vi "JKI_Python_Server - VI Tree.vi"   [LabVIEW 2013]
uses:
  Server/Server.lvclass
  Call/Call.lvclass
types:
  T1 = typedef "JKI_Python_Bridge_for_LV.lvlib/Server.lvclass/Python Method Call - Event Registration.ctl" = refnum<event-registration>
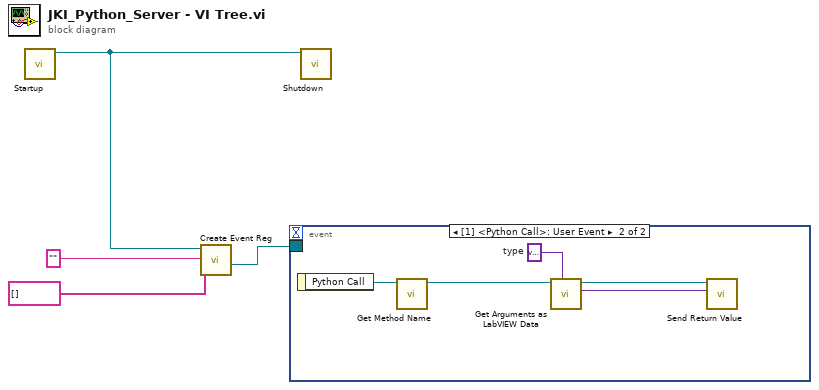
[diagram p0: block diagram]
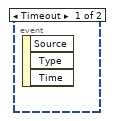
[diagram p2: hidden frame]
diagram:
  n1 = call "Startup.vi"() -> ("JKI_Python_Server out"=w4:refnum<class "Server.lvclass">)  [unwired: 10 in, 1 out]
  n2 = call "Create Event Reg.vi"("Method Names"=string[] [], "Object Name"="", "JKI_Python_Server in"=w4) -> ("Python"=w3:T1)  [unwired: 6 in, 2 out]
  n3 = event shown="[1] <Python Call>: User Event" {
    selector: w3 -> [_ _]
    dyn-events: _ -> [_ _]
    timeout: _ -> [_ _]
    event Timeout {
      n4 = event-data() -> ()  [unwired: 1 in, 3 out]
    }
    event User Event {
      w6 = variant  # type
      n5 = event-data() -> ("Python Call"=w9:refnum<class "Call.lvclass">)  [unwired: 1 in]
      n6 = call "Get Method Name.vi"("Call in"=w9) -> ("Call out"=w8:refnum<class "Call.lvclass">)  [unwired: 7 in, 3 out]
      n7 = call "Get Arguments as LabVIEW Data.vi"("type"=w6, "Call in"=w8) -> ("LabVIEW Data"=w5:variant, "Call out"=w7:refnum<class "Call.lvclass">)  [unwired: 7 in, 1 out]
      n8 = call "Send Return Value.vi"("Return Value"=w5, "Response in"=w7) -> ()  [unwired: 9 in, 1 out]
    }
  }
  n9 = call "Shutdown.vi"("JKI_Python_Server in"=w4) -> ()  [unwired: 10 in, 1 out]
